vi "CSMKVMap-InitDefaultValues.vi"(8 "error in":errorcluster) -> (0 "error out":errorcluster, 3 "KVMap":variant)   [LabVIEW 2017, in "Communicable State Machine.lvlib"]
uses:
  Communicable State Machine.lvlib
  CSMQ/_CSMOFGV.vi
  FGV-BroadcastRegistry/FGV-BroadcastRegistry.vi
  GlobalEvent/FGV-GlobalEventRef.vi
  GlobalEvent/FGV-GlobalEventQueues.vi
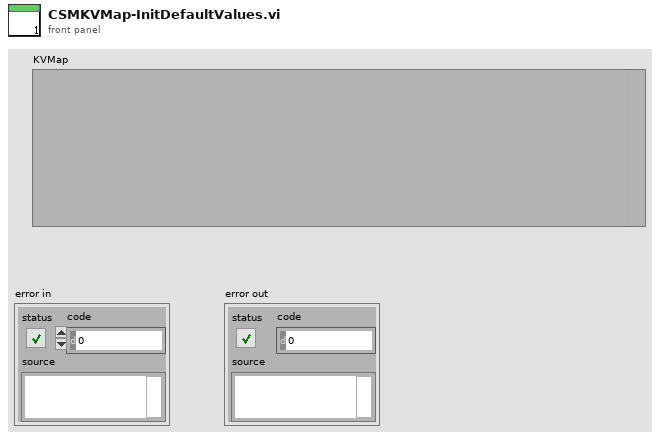
[diagram p1: front panel]
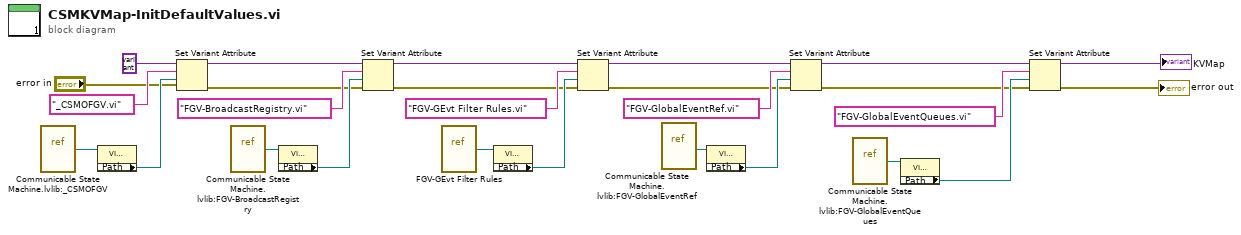
[diagram p0: block diagram]
diagram:
  n1 = vi-ref "Communicable State Machine.lvlib:_CSMOFGV.vi"() -> (w27:refnum<vi>)
  n2 = property class="VI (strict)"(reference=w27) -> ("Path"=w26:path)  [unwired: 1 in, 2 out]
  n3 = Set Variant Attribute(Variant=variant ("variant"), name="_CSMOFGV.vi", value=w26, error in="error in") -> (Variant out=w23:variant, error out=w6:errorcluster)  [unwired: 1 out]
  n4 = vi-ref "Communicable State Machine.lvlib:FGV-BroadcastRegistry.vi"() -> (w22:refnum<vi>)
  n5 = property class="VI (strict)"(reference=w22) -> ("Path"=w20:path)  [unwired: 1 in, 2 out]
  n6 = Set Variant Attribute(Variant=w23, name="FGV-BroadcastRegistry.vi", value=w20, error in=w6) -> (Variant out=w17:variant, error out=w5:errorcluster)  [unwired: 1 out]
  n7 = vi-ref "FGV-GEvt Filter Rules.vi"() -> (w16:refnum<vi>)
  n8 = property class="VI (strict)"(reference=w16) -> ("Path"=w19:path)  [unwired: 1 in, 2 out]
  n9 = Set Variant Attribute(Variant=w17, name="FGV-GEvt Filter Rules.vi", value=w19, error in=w5) -> (Variant out=w15:variant, error out=w4:errorcluster)  [unwired: 1 out]
  n10 = vi-ref "Communicable State Machine.lvlib:FGV-GlobalEventRef.vi"() -> (w12:refnum<vi>)
  n11 = property class="VI (strict)"(reference=w12) -> ("Path"=w13:path)  [unwired: 1 in, 2 out]
  n12 = Set Variant Attribute(Variant=w15, name="FGV-GlobalEventRef.vi", value=w13, error in=w4) -> (Variant out=w11:variant, error out=w3:errorcluster)  [unwired: 1 out]
  n13 = vi-ref "Communicable State Machine.lvlib:FGV-GlobalEventQueues.vi"() -> (w10:refnum<vi>)
  n14 = property class="VI (strict)"(reference=w10) -> ("Path"=w9:path)  [unwired: 1 in, 2 out]
  n15 = Set Variant Attribute(Variant=w11, name="FGV-GlobalEventQueues.vi", value=w9, error in=w3) -> (Variant out=→"KVMap":variant, error out=→"error out":errorcluster)  [unwired: 1 out]
